vi "Convert_1SDI_v00.vi"(8 "Extras PII":T1, 11 "PII Control":T2={"Offset Error"=-0.08983050847457627, "Gain Error"=1, "P Gain"=0, "P Bit Shift"=1, "I Bit Shift"=20, "I Gain"=-12, "Lock Threshold"=-12, "Lock"=FALSE, "Hold"=FALSE, "Scan Frequency"=8, "Scan Bit Shift"=-5, "Gains +/- "=TRUE, "Pre- Offset Error"=-5.0} {"Pre- Offset Error" scale=-0.01..0.01 scale format="%#_5f"; "Scan Frequency" scale=1.0..30.0; "I Gain" scale=0.0..50.0; "P Gain" scale=0.0..50.0; "Offset Error" scale=-0.01..0.01 scale format="%#_5f"}) -> (3 "PII+Error":T10)   [LabVIEW 2013]
uses:
  Strict Type Defs/PII individual.ctl
  Strict Type Defs/Errors Converted Graph.ctl
  Strict Type Defs/PII and Error Graph.ctl
  Strict Type Defs/Control GUI 1SDI EPR.ctl
  Strict Type Defs/Slider and display.ctl
  Strict Type Defs/I16 white control.ctl
  Strict Type Defs/PII Gains.ctl
  Strict Type Defs/Thresh slider.ctl
  Strict Type Defs/Lock or Hold.ctl
  Strict Type Defs/Scan Freq Slider.ctl
  Strict Type Defs/Gains negative horizontal.ctl
  Strict Type Defs/Extras PII 1SDI.ctl
panel:
  in  "PII+Error":T10
  in  "Error individual":T11
  in  "PII In typdef":T12
  # "Error Signal"
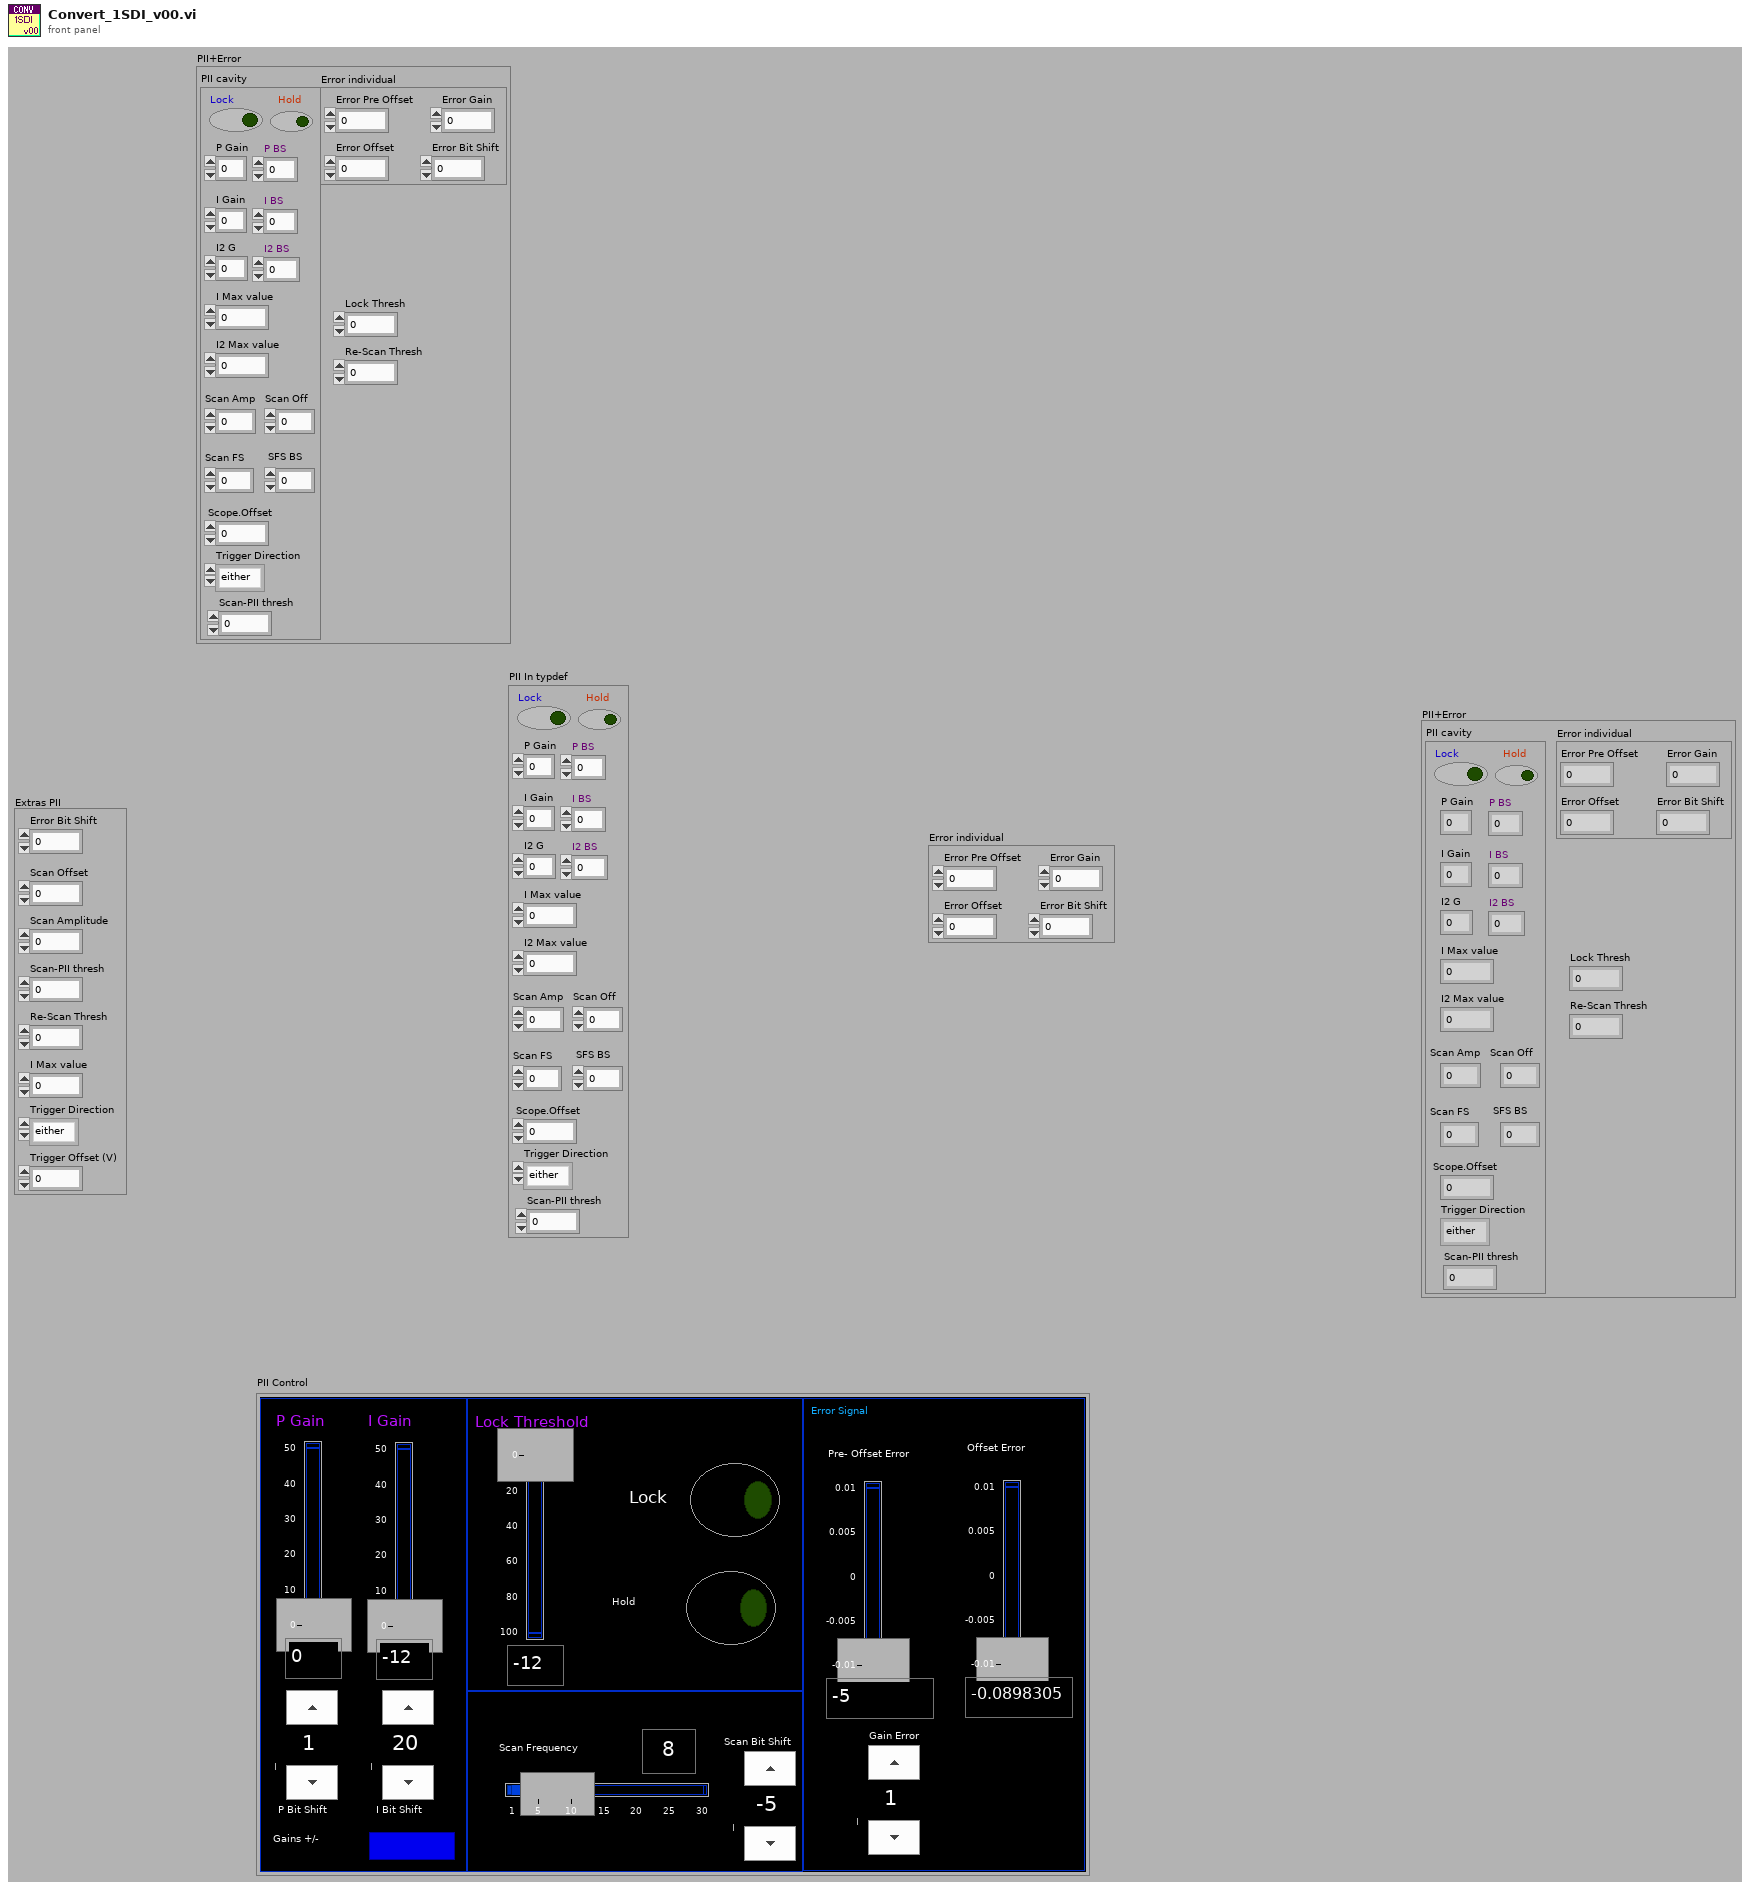
[diagram p1: front panel]
types:
  T1 = typedef "Extras PII 1SDI.ctl" = cluster{"Error Bit Shift":i16, "Scan Offset":dbl, "Scan Amplitude":dbl, "Scan-PII thresh":i16, "Re-Scan Thresh":i16, "I Max value":i32, "Trigger Direction":enum8{"either", "minus-plus", "plus-minus"}, "Trigger Offset (V)":dbl}
  T2 = typedef "Control GUI 1SDI EPR.ctl" = cluster{"Offset Error":T3, "Gain Error":T4, "P Gain":T5, "P Bit Shift":T4, "I Bit Shift":T4, "I Gain":T5, "Lock Threshold":T6, "Lock":T7, "Hold":T7, "Scan Frequency":T8, "Scan Bit Shift":T4, "Gains +/- ":T9, "Pre- Offset Error":T3}
  T3 = typedef "Slider and display.ctl" = dbl
  T4 = typedef "I16 white control.ctl" = i16
  T5 = typedef "PII Gains.ctl" = i32
  T6 = typedef "Thresh slider.ctl" = i16
  T7 = typedef "Lock or Hold.ctl" = bool
  T8 = typedef "Scan Freq Slider.ctl" = u16
  T9 = typedef "Gains negative horizontal.ctl" = bool
  T10 = typedef "PII and Error Graph.ctl" = cluster{"Error individual":T11, "PII cavity":T12, "Lock Thresh":i16, "Re-Scan Thresh":i16}
  T11 = typedef "Errors Converted Graph.ctl" = cluster{"Error Pre Offset":i16, "Error Offset":i16, "Error Gain":i16, "Error Bit Shift":i16}
  T12 = typedef "PII individual.ctl" = cluster{"Lock":bool, "Hold":bool, "P Gain":i32, "P BS":i16, "I Gain":i32, "I BS":i16, "I2 G":i32, "I2 BS":i16, "Scan Amp":i16, "Scan Off":i16, "Scan FS":u16, "SFS BS":i16, "I Max value":i32, "I2 Max value":i32, "Scope.Offset":i16, "Trigger Direction":enum8{"either", "minus-plus", "plus-minus"}, "Scan-PII thresh":i16}
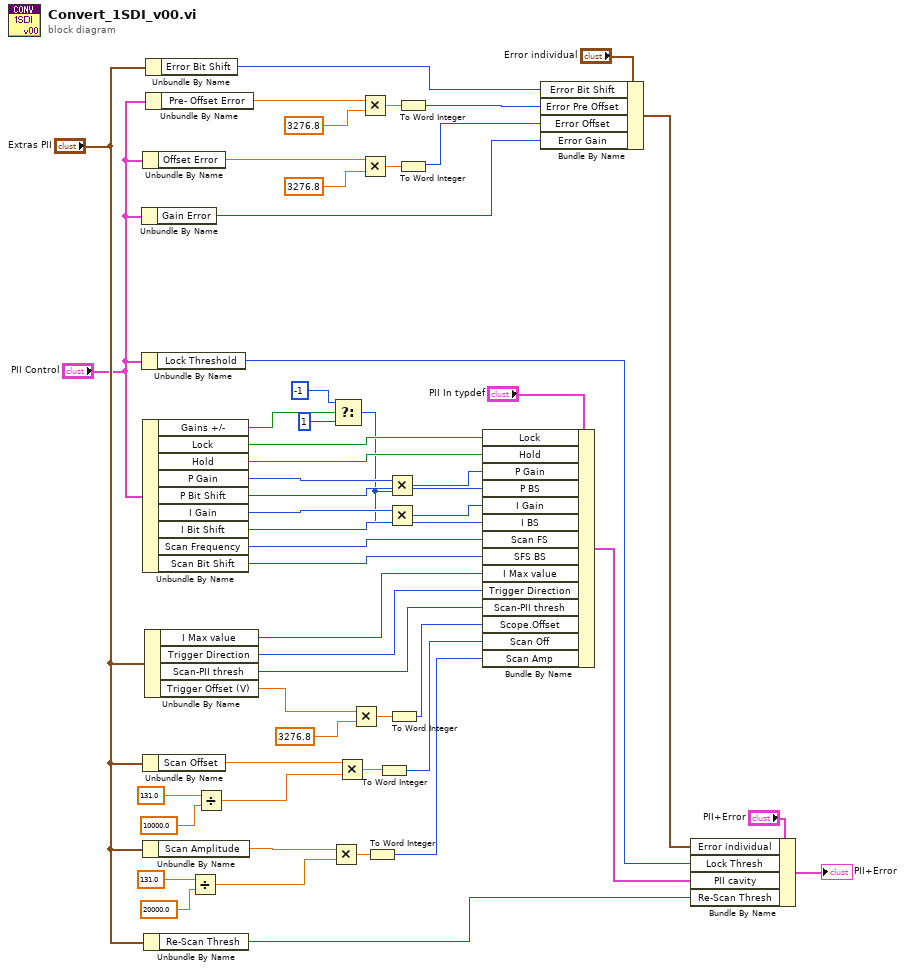
[diagram p0: block diagram]
diagram:
  n1 = Unbundle By Name("PII Control") -> ("Gain Error"=w19:T4)
  n2 = Unbundle By Name("PII Control") -> ("Lock Threshold"=w16:T6)
  n3 = Unbundle By Name("PII Control") -> ("Offset Error"=w49:T3)
  n4 = Unbundle By Name("PII Control") -> ("Gains +/-"=w34:T9, "Lock"=w38:T7, "Hold"=w37:T7, "P Gain"=w33:T5, "P Bit Shift"=w36:T4, "I Gain"=w29:T5, "I Bit Shift"=w35:T4, "Scan Frequency"=w26:T8, "Scan Bit Shift"=w25:T4)
  n5 = Unbundle By Name("Extras PII") -> ("Scan Offset"=w17:dbl)
  n6 = Unbundle By Name("Extras PII") -> ("Scan Amplitude"=w48:dbl)
  n7 = Unbundle By Name("Extras PII") -> ("Re-Scan Thresh"=w5:i16)
  n8 = Unbundle By Name("Extras PII") -> ("I Max value"=w13:i32, "Trigger Direction"=w12:enum8{"either", "minus-plus", "plus-minus"}, "Scan-PII thresh"=w11:i16, "Trigger Offset (V)"=w7:dbl)
  n9 = Unbundle By Name("Extras PII") -> ("Error Bit Shift"=w1:i16)
  n10 = Unbundle By Name("PII Control") -> ("Pre- Offset Error"=w2:T3)
  n11 = Divide(x=131.0, y=20000.0) -> (x/y=w43:dbl)
  n12 = Divide(x=131.0, y=10000.0) -> (x/y=w40:dbl)
  n13 = Multiply(x=w48, y=w43) -> (x*y=w46:dbl)
  n14 = Select(t=T5 -1 ("y"), s=w34, f=T5 1) -> (s? t:f=w27:T5)
  n15 = Multiply(x=w17, y=w40) -> (x*y=w47:dbl)
  n16 = Multiply(x=w7, y=3276.8) -> (x*y=w9:dbl)
  n17 = Multiply(x=w2, y=3276.8) -> (x*y=w52:T3)
  n18 = Multiply(x=w49, y=3276.8) -> (x*y=w51:T3)
  n19 = To Word Integer(number=w46) -> (16bit integer=w15:i16)
  n20 = To Word Integer(number=w47) -> (16bit integer=w10:i16)
  n21 = Multiply(x=w33, y=w27) -> (x*y=w30:T5)
  n22 = Multiply(x=w29, y=w27) -> (x*y=w28:T5)
  n23 = To Word Integer(number=w9) -> (16bit integer=w6:i16)
  n24 = To Word Integer(number=w52) -> (16bit integer=w23:i16)
  n25 = To Word Integer(number=w51) -> (16bit integer=w22:i16)
  n26 = Bundle By Name(cluster="PII In typdef", "Lock"=w38, "Hold"=w37, "P Gain"=w30, "P BS"=w36, "I Gain"=w28, "I BS"=w35, "Scan FS"=w26, "SFS BS"=w25, "I Max value"=w13, "Trigger Direction"=w12, "Scan-PII thresh"=w11, "Scope.Offset"=w6, "Scan Off"=w10, "Scan Amp"=w15) -> (w20:T12)
  n27 = Bundle By Name(cluster="Error individual", "Error Bit Shift"=w1, "Error Pre Offset"=w23, "Error Offset"=w22, "Error Gain"=w19) -> (w4:T11)
  n28 = Bundle By Name(cluster="PII+Error", "Error individual"=w4, "Lock Thresh"=w16, "PII cavity"=w20, "Re-Scan Thresh"=w5) -> (→"PII+Error":T10)
